vi "ResultSolver.vi"(8 "error in (no error)":errorcluster, 9 "Conf. Gral.":T2, 10 "Tipo de Med":T1, 11 "Array":sgl[](array[numeric])) -> (0 "error out":errorcluster, 3 "Result":sgl)   [LabVIEW 2014, in "MathLoop.lvlib"]
doc: "Calcula todos los resultados de Tiempo Real y Post-proceso."
uses:
  MathLoop.lvlib
  TypeDefs/Conf. Gral.ctl
  TypeDefs/typeMed.ctl
  <vilib>/Analysis/baseanly.llb/Mean (DBL).vi
  <vilib>/Analysis/2dsp.llb/Real FFT.vi
  <vilib>/Analysis/2dsp.llb/Inverse Complex FFT.vi
  <vilib>/Analysis/NI_AALBase.lvlib
  <vilib>/Analysis/NI_AALPro.lvlib
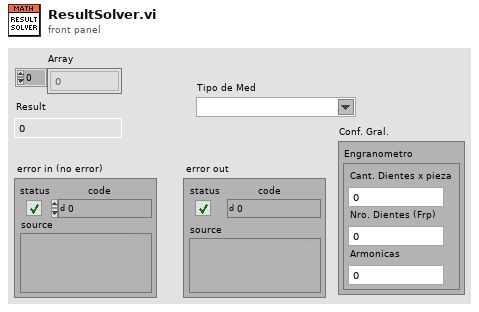
[diagram p1: front panel]
types:
  T1 = typedef "MathLoop.lvlib/typeMed.ctl" = string
  T2 = typedef "MathLoop.lvlib/Conf. Gral.ctl" = cluster{"Engranometro":cluster{"Cant. Dientes x pieza":i32, "Nro. Dientes (Frp)":i32, "Armonicas":i32}}
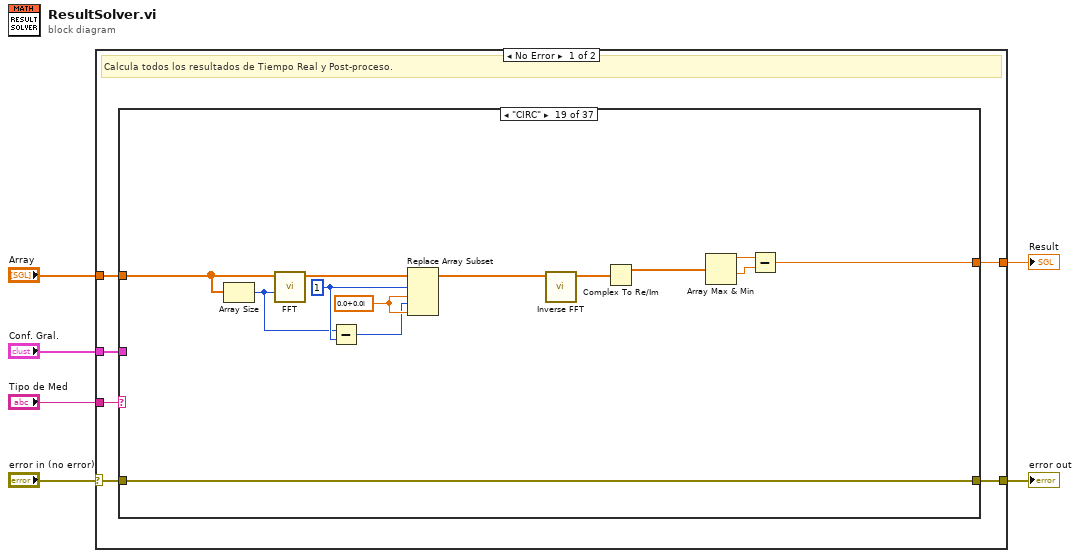
[diagram p0: block diagram]
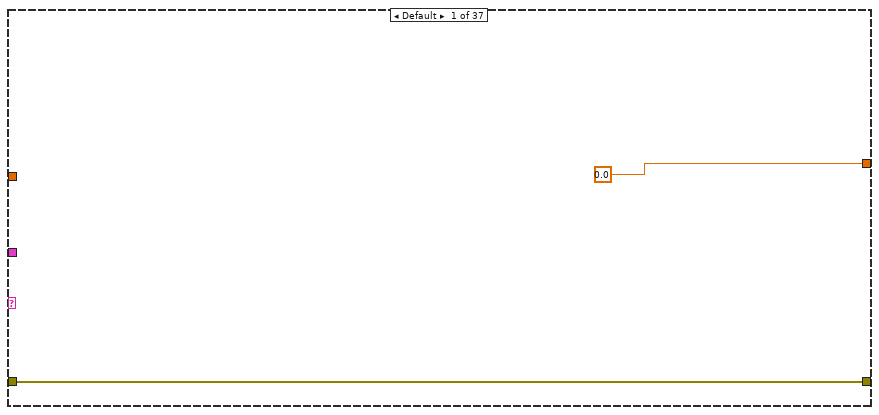
[diagram p2: hidden frame]
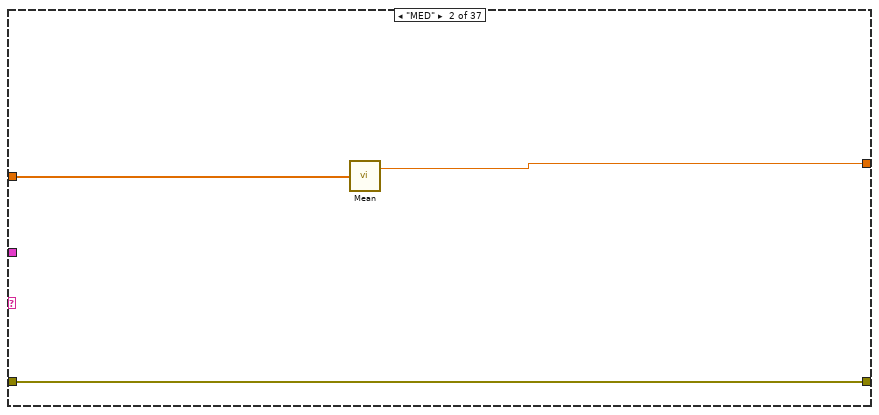
[diagram p3: hidden frame]
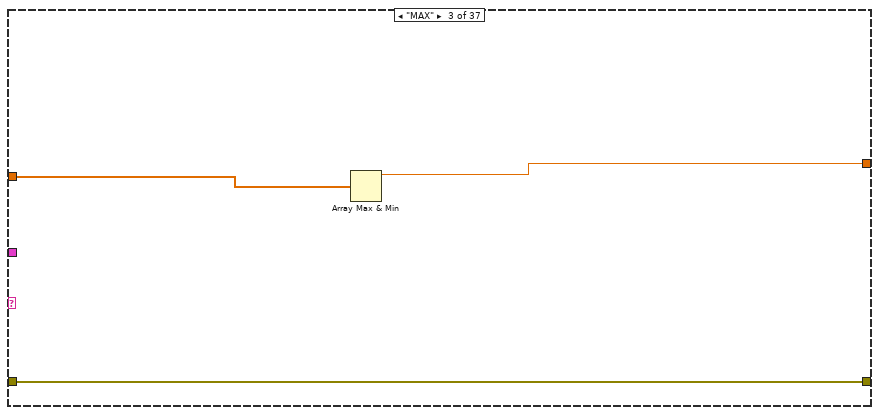
[diagram p4: hidden frame]
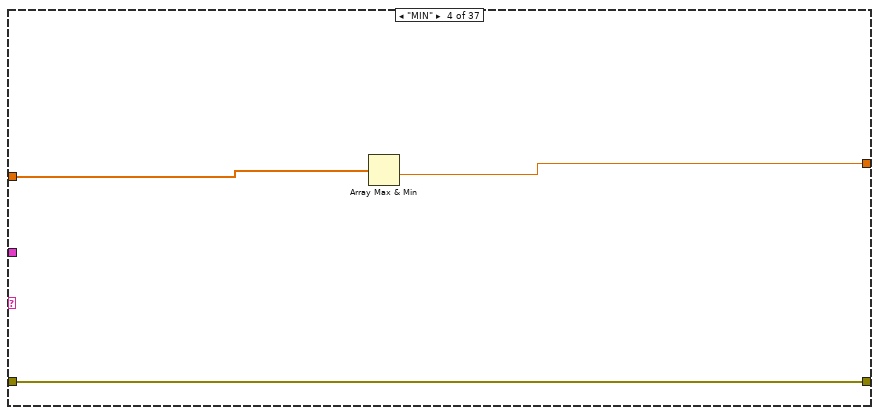
[diagram p5: hidden frame]
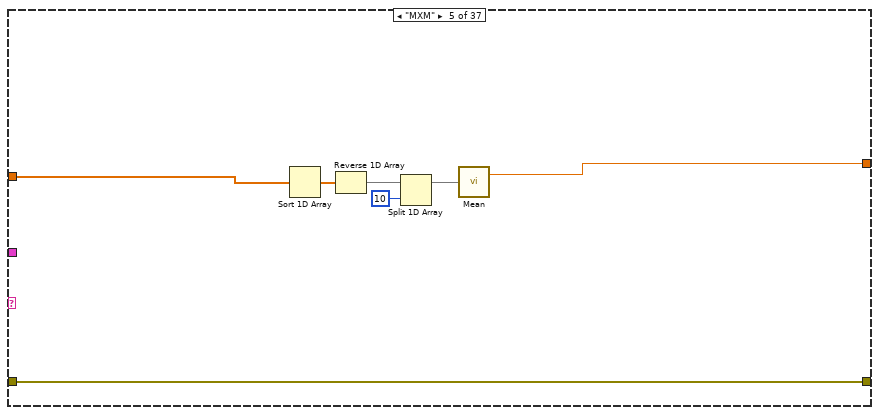
[diagram p6: hidden frame]
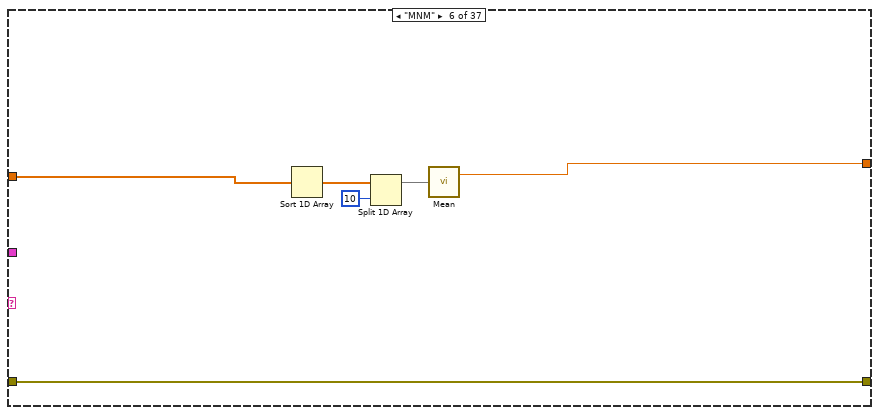
[diagram p7: hidden frame]
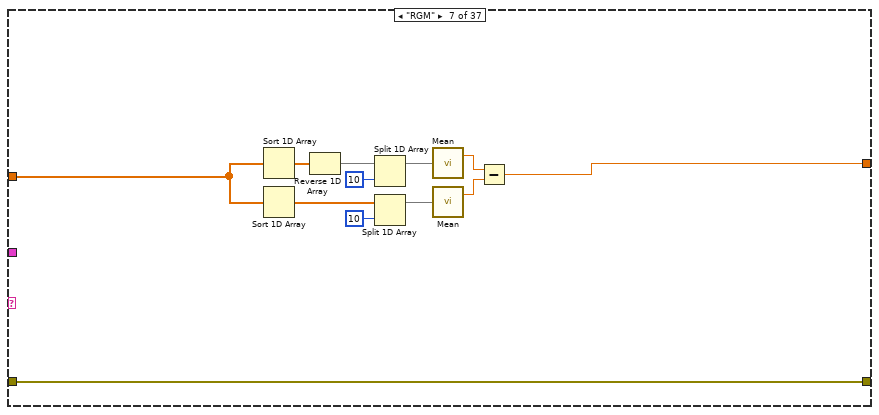
[diagram p8: hidden frame]
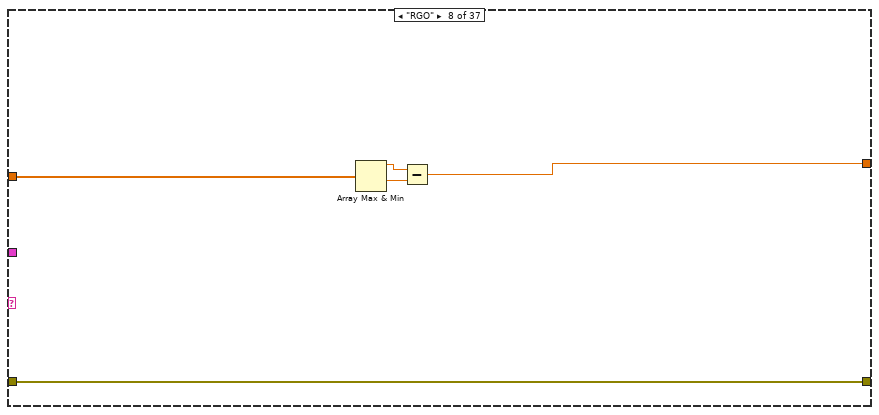
[diagram p9: hidden frame]
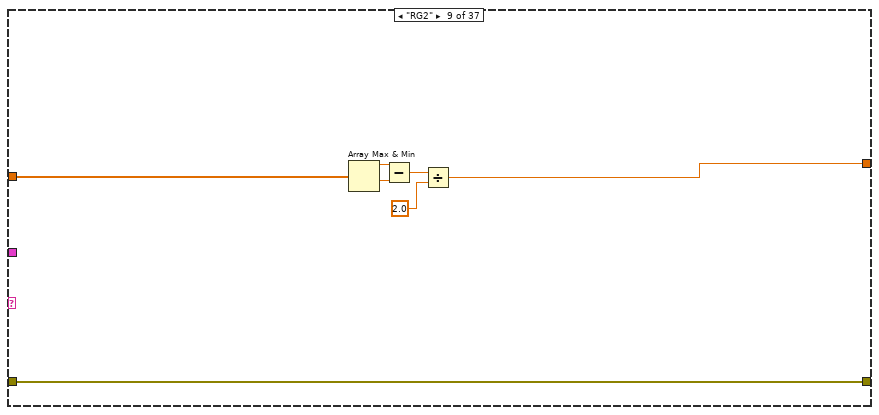
[diagram p10: hidden frame]
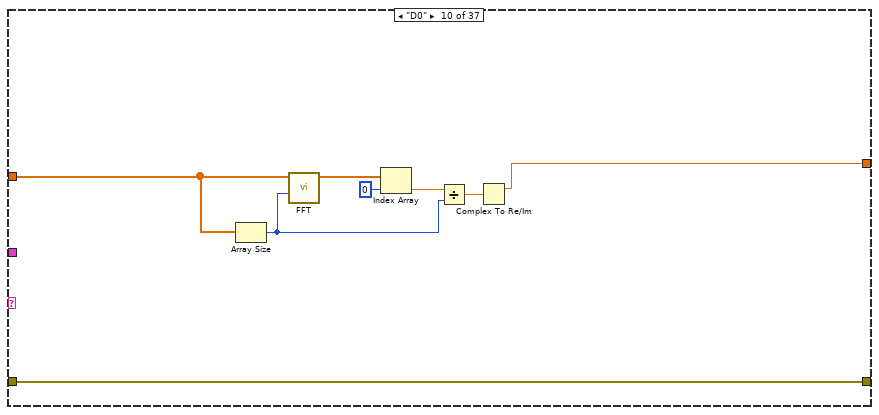
[diagram p11: hidden frame]
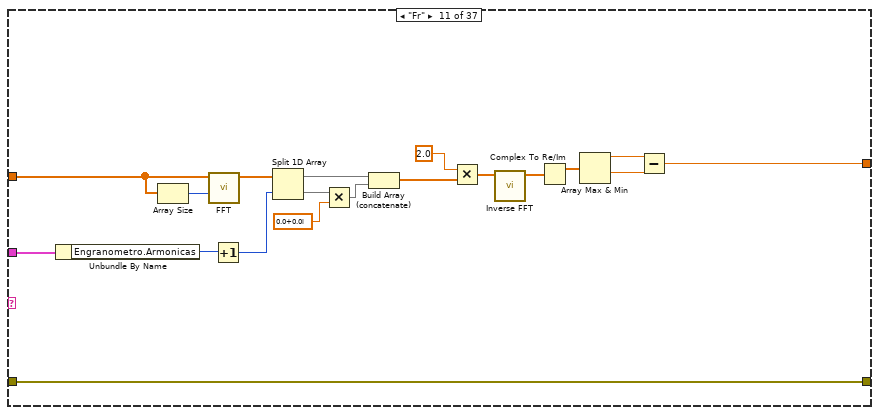
[diagram p12: hidden frame]
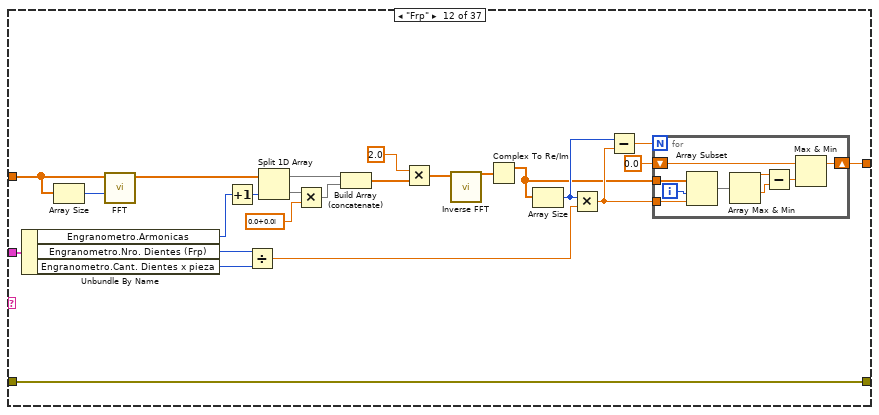
[diagram p13: hidden frame]
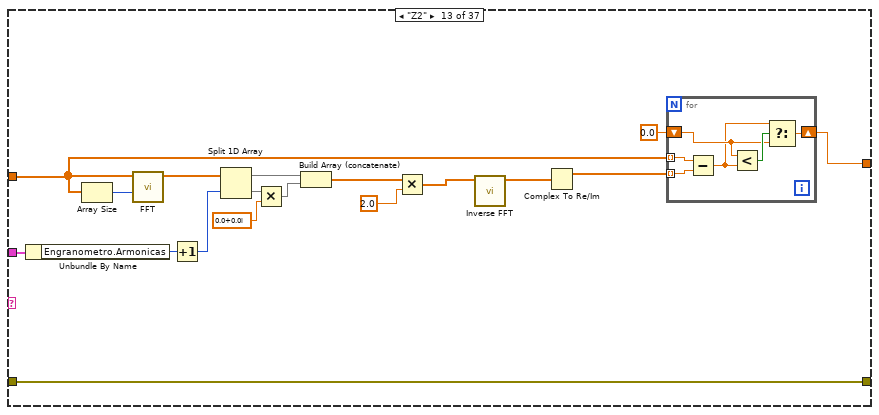
[diagram p14: hidden frame]
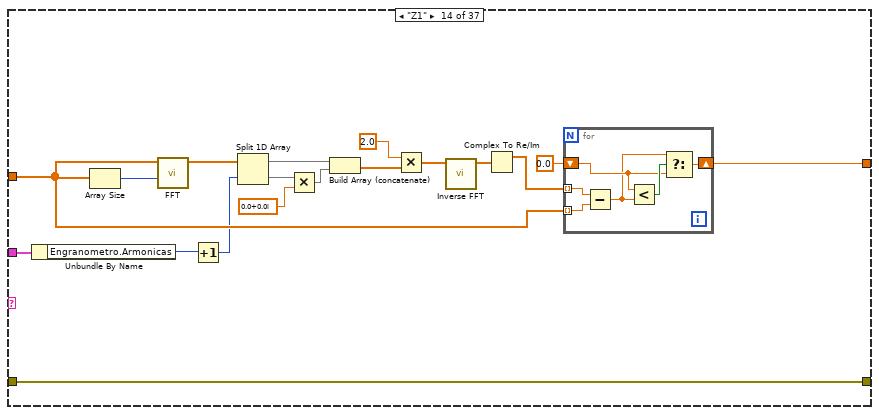
[diagram p15: hidden frame]
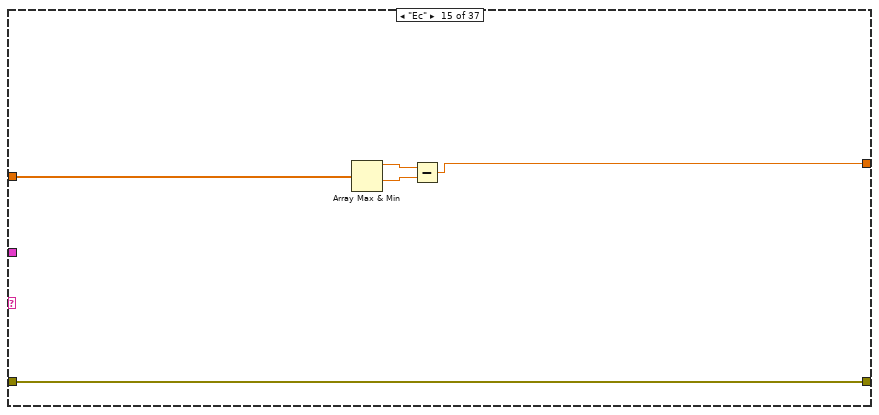
[diagram p16: hidden frame]
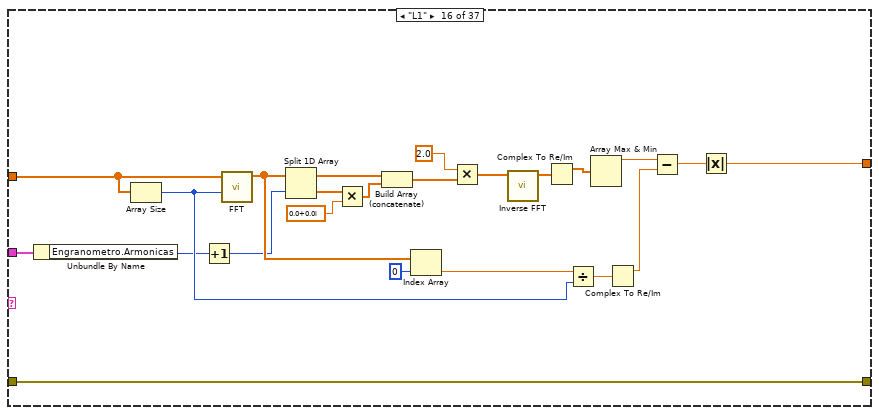
[diagram p17: hidden frame]
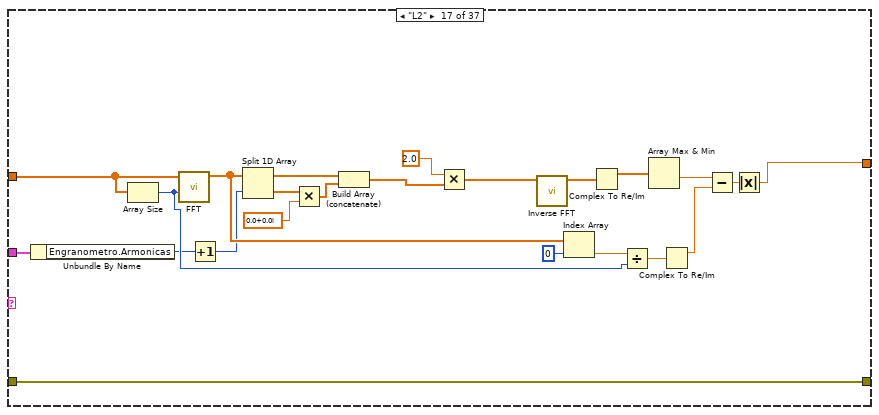
[diagram p18: hidden frame]
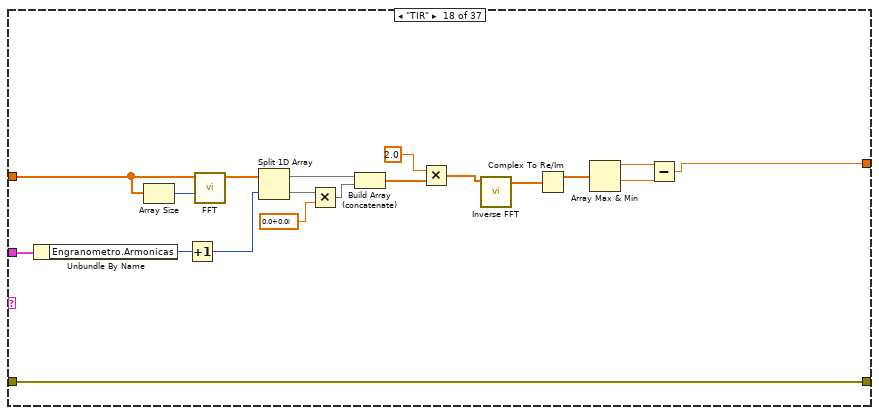
[diagram p19: hidden frame]
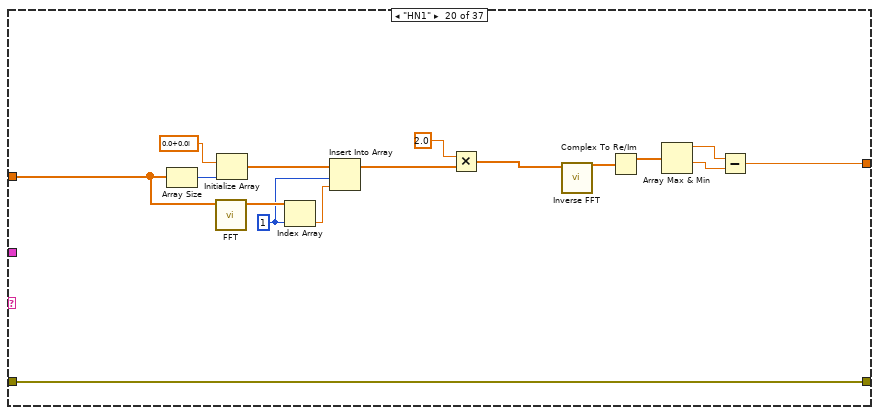
[diagram p20: hidden frame]
diagram:
  n1 = case shown="No Error" "error in (no error)" {
    selector: "error in (no error)" -> [w9 w561]
    tunnel: [w10 w561] -> w5
    tunnel: "Tipo de Med" -> [w12 _]
    tunnel: "Array" -> [w11 _]
    tunnel: [w7 0.0 ("mean")] -> w3
    tunnel: "Conf. Gral." -> [w8 _]
    frame No Error {
      # "Calcula todos los resultados de Tiempo Real y Post-proceso."
      n2 = case shown="\"CIRC\"" w12 {
        tunnel: w11 -> [_ w17 w20 w23 w25 w34 w40 w50 w59 w64 w86 w104 w130 w152 w172 w191 w214 w229 w247 w262 w274 w290 w306 w322 w338 w354 w370 w386 w402 w418 w434 w450 w466 w482 w498 w512 w554]
        tunnel: [0.0 ("mean") w16 w19 w22 w26 w33 w39 w51 w58 w61 w82 w95 w128 w153 w169 w181 w204 w228 w248 w258 w273 w289 w305 w321 w337 w353 w369 w385 w401 w417 w433 w449 w465 w481 w497 w510 w538] -> w7
        tunnel: [w14 w15 w18 w21 w24 w31 w38 w49 w54 w66 w87 w111 w138 w162 w173 w196 w219 w238 w251 w267 w283 w299 w315 w331 w347 w363 w379 w395 w411 w427 w443 w459 w475 w491 w507 w515 w559] -> w10
        tunnel: w9 -> [w14 w15 w18 w21 w24 w31 w38 w49 w54 w66 w87 w111 w138 w162 w173 w196 w219 w238 w251 w267 w283 w299 w315 w331 w347 w363 w379 w395 w411 w427 w443 w459 w475 w491 w507 w515 w559]
        tunnel: w8 -> [_ _ _ _ _ _ _ _ _ _ w81 w103 w131 w155 _ w190 w213 w227 _ _ _ _ _ _ _ _ _ _ _ _ _ _ _ _ _ w514 w555]
        frame Default {
        }
        frame "MED" {
          n3 = call-poly <vilib>:"Mean.vi"("X"=w17) -> ("mean"=w16:dbl)  [unwired: 1 out]
        }
        frame "MAX" {
          n4 = Array Max & Min(array=w20) -> (max value=w19:sgl)  [unwired: 3 out]
        }
        frame "MIN" {
          n5 = Array Max & Min(array=w23) -> (min value=w22:sgl)  [unwired: 3 out]
        }
        frame "MXM" {
          n6 = Sort 1D Array(array=w25) -> (sorted array=w28:sgl[])
          n7 = Reverse 1D Array(array=w28) -> (reversed array=w27:sgl[])
          n8 = Split 1D Array(array=w27, index=10) -> (first subarray=w29:sgl[])  [unwired: 1 out]
          n9 = call-poly <vilib>:"Mean.vi"("X"=w29) -> ("mean"=w26:dbl)  [unwired: 1 out]
        }
        frame "MNM" {
          n10 = Sort 1D Array(array=w34) -> (sorted array=w35:sgl[])
          n11 = Split 1D Array(array=w35, index=10) -> (first subarray=w36:sgl[])  [unwired: 1 out]
          n12 = call-poly <vilib>:"Mean.vi"("X"=w36) -> ("mean"=w33:dbl)  [unwired: 1 out]
        }
        frame "RGM" {
          n13 = Sort 1D Array(array=w40) -> (sorted array=w45:sgl[])
          n14 = Sort 1D Array(array=w40) -> (sorted array=w48:sgl[])
          n15 = Reverse 1D Array(array=w45) -> (reversed array=w46:sgl[])
          n16 = Split 1D Array(array=w46, index=10) -> (first subarray=w44:sgl[])  [unwired: 1 out]
          n17 = Split 1D Array(array=w48, index=10) -> (first subarray=w47:sgl[])  [unwired: 1 out]
          n18 = call-poly <vilib>:"Mean.vi"("X"=w44) -> ("mean"=w42:dbl)  [unwired: 1 out]
          n19 = call-poly <vilib>:"Mean.vi"("X"=w47) -> ("mean"=w41:dbl)  [unwired: 1 out]
          n20 = Subtract(x=w42, y=w41) -> (x-y=w39:dbl)
        }
        frame "RGO" {
          n21 = Array Max & Min(array=w50) -> (max value=w53:sgl, min value=w52:sgl)  [unwired: 2 out]
          n22 = Subtract(x=w53, y=w52) -> (x-y=w51:sgl)
        }
        frame "RG2" {
          n23 = Array Max & Min(array=w59) -> (max value=w56:sgl, min value=w55:sgl)  [unwired: 2 out]
          n24 = Subtract(x=w56, y=w55) -> (x-y=w57:sgl)
          n25 = Divide(x=w57, y=sgl 2.0) -> (x/y=w58:sgl)
        }
        frame "D0" {
          n26 = Array Size(array=w64) -> (size(s)=w63:i32)
          n27 = call-poly <vilib>:"FFT.vi"("FFT size"=w63, "X"=w64) -> ("FFT {X}"=w68:cdb[])  [unwired: 8 in, 1 out]
          n28 = Index Array(array=w68, index=0) -> (element=w62:cdb)
          n29 = Divide(x=w62, y=w63) -> (x/y=w65:cdb)
          n30 = Complex To Re/Im(x + iy=w65) -> (x=w61:dbl)  [unwired: 1 out]
        }
        frame "Fr" {
          n31 = Unbundle By Name(w81) -> ("Engranometro.Armonicas"=w73:i32)
          n32 = Array Size(array=w86) -> (size(s)=w85:i32)
          n33 = call-poly <vilib>:"FFT.vi"("FFT size"=w85, "X"=w86) -> ("FFT {X}"=w80:cdb[])  [unwired: 8 in, 1 out]
          n34 = Increment(x=w73) -> (x+1=w72:i32)
          n35 = Split 1D Array(array=w80, index=w72) -> (first subarray=w79:cdb[], second subarray=w76:cdb[])
          n36 = Multiply(x=w76, y=cdb 0.0+0.0i) -> (x*y=w77:cdb[])
          n37 = Build Array (concatenate)(w79, w77) -> (w70:cdb[])
          n38 = Multiply(x=2.0, y=w70) -> (x*y=w69:cdb[])
          n39 = call-poly <vilib>:"Inverse FFT.vi"("FFT {X}"=w69) -> ("X"=w75:cdb[])  [unwired: 9 in, 1 out]
          n40 = Complex To Re/Im(x + iy=w75) -> (x=w74:dbl[])  [unwired: 1 out]
          n41 = Array Max & Min(array=w74) -> (max value=w84:dbl, min value=w83:dbl)  [unwired: 2 out]
          n42 = Subtract(x=w84, y=w83) -> (x-y=w82:dbl)
        }
        frame "Frp" {
          n43 = Unbundle By Name(w103) -> ("Engranometro.Armonicas"=w91:i32, "Engranometro.Nro. Dientes (Frp)"=w98:i32, "Engranometro.Cant. Dientes x pieza"=w97:i32)
          n44 = Array Size(array=w104) -> (size(s)=w110:i32)
          n45 = call-poly <vilib>:"FFT.vi"("FFT size"=w110, "X"=w104) -> ("FFT {X}"=w109:cdb[])  [unwired: 8 in, 1 out]
          n46 = Increment(x=w91) -> (x+1=w92:i32)
          n47 = Divide(x=w98, y=w97) -> (x/y=w96:dbl)
          n48 = Split 1D Array(array=w109, index=w92) -> (first subarray=w108:cdb[], second subarray=w105:cdb[])
          n49 = Multiply(x=w105, y=cdb 0.0+0.0i) -> (x*y=w106:cdb[])
          n50 = Build Array (concatenate)(w108, w106) -> (w89:cdb[])
          n51 = Multiply(x=2.0, y=w89) -> (x*y=w88:cdb[])
          n52 = call-poly <vilib>:"Inverse FFT.vi"("FFT {X}"=w88) -> ("X"=w94:cdb[])  [unwired: 9 in, 1 out]
          n53 = Complex To Re/Im(x + iy=w94) -> (x=w93:dbl[])  [unwired: 1 out]
          n54 = Array Size(array=w93) -> (size(s)=w101:i32)
          n55 = Multiply(x=w101, y=w96) -> (x*y=w100:dbl)
          n56 = Subtract(x=w101, y=w100) -> (x-y=w99:dbl)
          n57 = for {
            N: w99 -> [_]
            tunnel: w93 -> [w114]
            tunnel: w100 -> [w113]
            shift-right: [w117] -> w95
            shift-left: 0.0 ("element") -> [w115]
            i -> [w112]
            n58 = Array Subset(array=w114, index=w112, length=w113) -> (w120:dbl[])
            n59 = Array Max & Min(array=w120) -> (max value=w119:dbl, min value=w118:dbl)  [unwired: 2 out]
            n60 = Subtract(x=w119, y=w118) -> (x-y=w116:dbl)
            n61 = Max & Min(x=w115, y=w116) -> (max(x,y)=w117:dbl)  [unwired: 1 out]
          }
        }
        frame "Z2" {
          n62 = Unbundle By Name(w131) -> ("Engranometro.Armonicas"=w125:i32)
          n63 = Array Size(array=w130) -> (size(s)=w137:i32)
          n64 = call-poly <vilib>:"FFT.vi"("FFT size"=w137, "X"=w130) -> ("FFT {X}"=w136:cdb[])  [unwired: 8 in, 1 out]
          n65 = Increment(x=w125) -> (x+1=w124:i32)
          n66 = Split 1D Array(array=w136, index=w124) -> (first subarray=w135:cdb[], second subarray=w132:cdb[])
          n67 = Multiply(x=w132, y=cdb 0.0+0.0i) -> (x*y=w133:cdb[])
          n68 = Build Array (concatenate)(w135, w133) -> (w121:cdb[])
          n69 = Multiply(x=w121, y=2.0 ("x")) -> (x*y=w122:cdb[])
          n70 = call-poly <vilib>:"Inverse FFT.vi"("FFT {X}"=w122) -> ("X"=w127:cdb[])  [unwired: 9 in, 1 out]
          n71 = Complex To Re/Im(x + iy=w127) -> (x=w126:dbl[])  [unwired: 1 out]
          n72 = for {
            tunnel: w126 -> [w143] mode=indexing
            tunnel: w130 -> [w144] mode=indexing
            shift-right: [w139] -> w128
            shift-left: 0.0 -> [w141]
            n73 = Subtract(x=w144, y=w143) -> (x-y=w140:dbl)
            n74 = Less?(x=w141, y=w140) -> (x < y?=w142:bool)
            n75 = Select(t=w140, s=w142, f=w141) -> (s? t:f=w139:dbl)
          }
        }
        frame "Z1" {
          n76 = Unbundle By Name(w155) -> ("Engranometro.Armonicas"=w149:i32)
          n77 = Array Size(array=w152) -> (size(s)=w161:i32)
          n78 = call-poly <vilib>:"FFT.vi"("FFT size"=w161, "X"=w152) -> ("FFT {X}"=w160:cdb[])  [unwired: 8 in, 1 out]
          n79 = Increment(x=w149) -> (x+1=w148:i32)
          n80 = Split 1D Array(array=w160, index=w148) -> (first subarray=w159:cdb[], second subarray=w156:cdb[])
          n81 = Multiply(x=w156, y=cdb 0.0+0.0i) -> (x*y=w157:cdb[])
          n82 = Build Array (concatenate)(w159, w157) -> (w146:cdb[])
          n83 = Multiply(x=2.0, y=w146) -> (x*y=w145:cdb[])
          n84 = call-poly <vilib>:"Inverse FFT.vi"("FFT {X}"=w145) -> ("X"=w151:cdb[])  [unwired: 9 in, 1 out]
          n85 = Complex To Re/Im(x + iy=w151) -> (x=w150:dbl[])  [unwired: 1 out]
          n86 = for {
            tunnel: w152 -> [w167] mode=indexing
            tunnel: w150 -> [w168] mode=indexing
            shift-right: [w163] -> w153
            shift-left: 0.0 -> [w165]
            n87 = Subtract(x=w168, y=w167) -> (x-y=w164:dbl)
            n88 = Less?(x=w165, y=w164) -> (x < y?=w166:bool)
            n89 = Select(t=w164, s=w166, f=w165) -> (s? t:f=w163:dbl)
          }
        }
        frame "Ec" {
          n90 = Array Max & Min(array=w172) -> (max value=w171:sgl, min value=w170:sgl)  [unwired: 2 out]
          n91 = Subtract(x=w171, y=w170) -> (x-y=w169:sgl)
        }
        frame "L1" {
          n92 = Unbundle By Name(w190) -> ("Engranometro.Armonicas"=w178:i32)
          n93 = Array Size(array=w191) -> (size(s)=w184:i32)
          n94 = Increment(x=w178) -> (x+1=w177:i32)
          n95 = call-poly <vilib>:"FFT.vi"("FFT size"=w184, "X"=w191) -> ("FFT {X}"=w185:cdb[])  [unwired: 8 in, 1 out]
          n96 = Split 1D Array(array=w185, index=w177) -> (first subarray=w195:cdb[], second subarray=w192:cdb[])
          n97 = Multiply(x=w192, y=cdb 0.0+0.0i) -> (x*y=w193:cdb[])
          n98 = Build Array (concatenate)(w195, w193) -> (w175:cdb[])
          n99 = Index Array(array=w185, index=0) -> (element=w186:cdb)
          n100 = Multiply(x=2.0, y=w175) -> (x*y=w174:cdb[])
          n101 = call-poly <vilib>:"Inverse FFT.vi"("FFT {X}"=w174) -> ("X"=w180:cdb[])  [unwired: 9 in, 1 out]
          n102 = Complex To Re/Im(x + iy=w180) -> (x=w179:dbl[])  [unwired: 1 out]
          n103 = Divide(x=w186, y=w184) -> (x/y=w187:cdb)
          n104 = Array Max & Min(array=w179) -> (max value=w189:dbl)  [unwired: 3 out]
          n105 = Complex To Re/Im(x + iy=w187) -> (x=w183:dbl)  [unwired: 1 out]
          n106 = Subtract(x=w189, y=w183) -> (x-y=w182:dbl)
          n107 = Absolute Value(x=w182) -> (abs(x)=w181:dbl)
        }
        frame "L2" {
          n108 = Unbundle By Name(w213) -> ("Engranometro.Armonicas"=w200:i32)
          n109 = Array Size(array=w214) -> (size(s)=w206:i32)
          n110 = call-poly <vilib>:"FFT.vi"("FFT size"=w206, "X"=w214) -> ("FFT {X}"=w207:cdb[])  [unwired: 8 in, 1 out]
          n111 = Increment(x=w200) -> (x+1=w201:i32)
          n112 = Split 1D Array(array=w207, index=w201) -> (first subarray=w218:cdb[], second subarray=w215:cdb[])
          n113 = Multiply(x=w215, y=cdb 0.0+0.0i) -> (x*y=w216:cdb[])
          n114 = Build Array (concatenate)(w218, w216) -> (w198:cdb[])
          n115 = Multiply(x=2.0, y=w198) -> (x*y=w197:cdb[])
          n116 = call-poly <vilib>:"Inverse FFT.vi"("FFT {X}"=w197) -> ("X"=w203:cdb[])  [unwired: 9 in, 1 out]
          n117 = Index Array(array=w207, index=0) -> (element=w210:cdb)
          n118 = Complex To Re/Im(x + iy=w203) -> (x=w202:dbl[])  [unwired: 1 out]
          n119 = Divide(x=w210, y=w206) -> (x/y=w211:cdb)
          n120 = Array Max & Min(array=w202) -> (min value=w209:dbl)  [unwired: 3 out]
          n121 = Complex To Re/Im(x + iy=w211) -> (x=w208:dbl)  [unwired: 1 out]
          n122 = Subtract(x=w209, y=w208) -> (x-y=w205:dbl)
          n123 = Absolute Value(x=w205) -> (abs(x)=w204:dbl)
        }
        frame "TIR" {
          n124 = Unbundle By Name(w227) -> ("Engranometro.Armonicas"=w224:i32)
          n125 = Array Size(array=w229) -> (size(s)=w237:i32)
          n126 = Increment(x=w224) -> (x+1=w223:i32)
          n127 = call-poly <vilib>:"FFT.vi"("FFT size"=w237, "X"=w229) -> ("FFT {X}"=w234:cdb[])  [unwired: 8 in, 1 out]
          n128 = Split 1D Array(array=w234, index=w223) -> (first subarray=w233:cdb[], second subarray=w230:cdb[])
          n129 = Multiply(x=w230, y=cdb 0.0+0.0i) -> (x*y=w231:cdb[])
          n130 = Build Array (concatenate)(w233, w231) -> (w221:cdb[])
          n131 = Multiply(x=2.0, y=w221) -> (x*y=w220:cdb[])
          n132 = call-poly <vilib>:"Inverse FFT.vi"("FFT {X}"=w220) -> ("X"=w226:cdb[])  [unwired: 9 in, 1 out]
          n133 = Complex To Re/Im(x + iy=w226) -> (x=w225:dbl[])  [unwired: 1 out]
          n134 = Array Max & Min(array=w225) -> (max value=w236:dbl, min value=w235:dbl)  [unwired: 2 out]
          n135 = Subtract(x=w236, y=w235) -> (x-y=w228:dbl)
        }
        frame "CIRC" {
          w244 = cdb 0.0+0.0i ("new element/subarray")
          w240 = 1 ("index")
          n136 = Array Size(array=w247) -> (size(s)=w239:i32)
          n137 = call-poly <vilib>:"FFT.vi"("FFT size"=w239, "X"=w247) -> ("FFT {X}"=w242:cdb[])  [unwired: 8 in, 1 out]
          n138 = Subtract(x=w239, y=w240) -> (x-y=w243:i32)
          n139 = Replace Array Subset(array=w242, new element #1=w244, index #1=w240, new element #2=w244, index #2=w243) -> (w241:cdb[])
          n140 = call-poly <vilib>:"Inverse FFT.vi"("FFT {X}"=w241) -> ("X"=w246:cdb[])  [unwired: 9 in, 1 out]
          n141 = Complex To Re/Im(x + iy=w246) -> (x=w245:dbl[])  [unwired: 1 out]
          n142 = Array Max & Min(array=w245) -> (max value=w250:dbl, min value=w249:dbl)  [unwired: 2 out]
          n143 = Subtract(x=w250, y=w249) -> (x-y=w248:dbl)
        }
        frame "HN1" {
          w261 = 1 ("index")
          n144 = Array Size(array=w262) -> (size(s)=w263:i32)
          n145 = call-poly <vilib>:"FFT.vi"("X"=w262) -> ("FFT {X}"=w264:cdb[])  [unwired: 9 in, 1 out]
          n146 = Initialize Array(cdb 0.0+0.0i ("element"), w263) -> (w266:cdb[])
          n147 = Index Array(array=w264, index=w261) -> (element=w257:cdb)
          n148 = Insert Into Array(array=w266, index=w261, new element=w257) -> (w253:cdb[])
          n149 = Multiply(x=2.0, y=w253) -> (x*y=w252:cdb[])
          n150 = call-poly <vilib>:"Inverse FFT.vi"("FFT {X}"=w252) -> ("X"=w256:cdb[])  [unwired: 9 in, 1 out]
          n151 = Complex To Re/Im(x + iy=w256) -> (x=w255:dbl[])  [unwired: 1 out]
          n152 = Array Max & Min(array=w255) -> (max value=w260:dbl, min value=w259:dbl)  [unwired: 2 out]
          n153 = Subtract(x=w260, y=w259) -> (x-y=w258:dbl)
        }
        frame "HN2" {
          w279 = 2 ("index")
          n154 = Array Size(array=w274) -> (size(s)=w278:i32)
          n155 = call-poly <vilib>:"FFT.vi"("X"=w274) -> ("FFT {X}"=w277:cdb[])  [unwired: 9 in, 1 out]
          n156 = Initialize Array(cdb 0.0+0.0i ("element"), w278) -> (w275:cdb[])
          n157 = Index Array(array=w277, index=w279) -> (element=w282:cdb)
          n158 = Insert Into Array(array=w275, index=w279, new element=w282) -> (w269:cdb[])
          n159 = Multiply(x=2.0, y=w269) -> (x*y=w268:cdb[])
          n160 = call-poly <vilib>:"Inverse FFT.vi"("FFT {X}"=w268) -> ("X"=w272:cdb[])  [unwired: 9 in, 1 out]
          n161 = Complex To Re/Im(x + iy=w272) -> (x=w271:dbl[])  [unwired: 1 out]
          n162 = Array Max & Min(array=w271) -> (max value=w280:dbl, min value=w281:dbl)  [unwired: 2 out]
          n163 = Subtract(x=w280, y=w281) -> (x-y=w273:dbl)
        }
        frame "HN3" {
          w295 = 3 ("index")
          n164 = Array Size(array=w290) -> (size(s)=w294:i32)
          n165 = call-poly <vilib>:"FFT.vi"("X"=w290) -> ("FFT {X}"=w293:cdb[])  [unwired: 9 in, 1 out]
          n166 = Initialize Array(cdb 0.0+0.0i ("element"), w294) -> (w291:cdb[])
          n167 = Index Array(array=w293, index=w295) -> (element=w298:cdb)
          n168 = Insert Into Array(array=w291, index=w295, new element=w298) -> (w285:cdb[])
          n169 = Multiply(x=2.0, y=w285) -> (x*y=w284:cdb[])
          n170 = call-poly <vilib>:"Inverse FFT.vi"("FFT {X}"=w284) -> ("X"=w288:cdb[])  [unwired: 9 in, 1 out]
          n171 = Complex To Re/Im(x + iy=w288) -> (x=w287:dbl[])  [unwired: 1 out]
          n172 = Array Max & Min(array=w287) -> (max value=w296:dbl, min value=w297:dbl)  [unwired: 2 out]
          n173 = Subtract(x=w296, y=w297) -> (x-y=w289:dbl)
        }
        frame "HN4" {
          w311 = 4 ("index")
          n174 = Array Size(array=w306) -> (size(s)=w310:i32)
          n175 = call-poly <vilib>:"FFT.vi"("X"=w306) -> ("FFT {X}"=w309:cdb[])  [unwired: 9 in, 1 out]
          n176 = Initialize Array(cdb 0.0+0.0i ("element"), w310) -> (w307:cdb[])
          n177 = Index Array(array=w309, index=w311) -> (element=w314:cdb)
          n178 = Insert Into Array(array=w307, index=w311, new element=w314) -> (w301:cdb[])
          n179 = Multiply(x=2.0, y=w301) -> (x*y=w300:cdb[])
          n180 = call-poly <vilib>:"Inverse FFT.vi"("FFT {X}"=w300) -> ("X"=w304:cdb[])  [unwired: 9 in, 1 out]
          n181 = Complex To Re/Im(x + iy=w304) -> (x=w303:dbl[])  [unwired: 1 out]
          n182 = Array Max & Min(array=w303) -> (max value=w312:dbl, min value=w313:dbl)  [unwired: 2 out]
          n183 = Subtract(x=w312, y=w313) -> (x-y=w305:dbl)
        }
        frame "HN5" {
          w327 = 5 ("index")
          n184 = Array Size(array=w322) -> (size(s)=w326:i32)
          n185 = call-poly <vilib>:"FFT.vi"("X"=w322) -> ("FFT {X}"=w325:cdb[])  [unwired: 9 in, 1 out]
          n186 = Initialize Array(cdb 0.0+0.0i ("element"), w326) -> (w323:cdb[])
          n187 = Index Array(array=w325, index=w327) -> (element=w330:cdb)
          n188 = Insert Into Array(array=w323, index=w327, new element=w330) -> (w317:cdb[])
          n189 = Multiply(x=2.0, y=w317) -> (x*y=w316:cdb[])
          n190 = call-poly <vilib>:"Inverse FFT.vi"("FFT {X}"=w316) -> ("X"=w320:cdb[])  [unwired: 9 in, 1 out]
          n191 = Complex To Re/Im(x + iy=w320) -> (x=w319:dbl[])  [unwired: 1 out]
          n192 = Array Max & Min(array=w319) -> (max value=w328:dbl, min value=w329:dbl)  [unwired: 2 out]
          n193 = Subtract(x=w328, y=w329) -> (x-y=w321:dbl)
        }
        frame "HN6" {
          w343 = 6 ("index")
          n194 = Array Size(array=w338) -> (size(s)=w342:i32)
          n195 = call-poly <vilib>:"FFT.vi"("X"=w338) -> ("FFT {X}"=w341:cdb[])  [unwired: 9 in, 1 out]
          n196 = Initialize Array(cdb 0.0+0.0i ("element"), w342) -> (w339:cdb[])
          n197 = Index Array(array=w341, index=w343) -> (element=w346:cdb)
          n198 = Insert Into Array(array=w339, index=w343, new element=w346) -> (w333:cdb[])
          n199 = Multiply(x=2.0, y=w333) -> (x*y=w332:cdb[])
          n200 = call-poly <vilib>:"Inverse FFT.vi"("FFT {X}"=w332) -> ("X"=w336:cdb[])  [unwired: 9 in, 1 out]
          n201 = Complex To Re/Im(x + iy=w336) -> (x=w335:dbl[])  [unwired: 1 out]
          n202 = Array Max & Min(array=w335) -> (max value=w344:dbl, min value=w345:dbl)  [unwired: 2 out]
          n203 = Subtract(x=w344, y=w345) -> (x-y=w337:dbl)
        }
        frame "HN7" {
          w359 = 7 ("index")
          n204 = Array Size(array=w354) -> (size(s)=w358:i32)
          n205 = call-poly <vilib>:"FFT.vi"("X"=w354) -> ("FFT {X}"=w357:cdb[])  [unwired: 9 in, 1 out]
          n206 = Initialize Array(cdb 0.0+0.0i ("element"), w358) -> (w355:cdb[])
          n207 = Index Array(array=w357, index=w359) -> (element=w362:cdb)
          n208 = Insert Into Array(array=w355, index=w359, new element=w362) -> (w349:cdb[])
          n209 = Multiply(x=2.0, y=w349) -> (x*y=w348:cdb[])
          n210 = call-poly <vilib>:"Inverse FFT.vi"("FFT {X}"=w348) -> ("X"=w352:cdb[])  [unwired: 9 in, 1 out]
          n211 = Complex To Re/Im(x + iy=w352) -> (x=w351:dbl[])  [unwired: 1 out]
          n212 = Array Max & Min(array=w351) -> (max value=w360:dbl, min value=w361:dbl)  [unwired: 2 out]
          n213 = Subtract(x=w360, y=w361) -> (x-y=w353:dbl)
        }
        frame "HN8" {
          w375 = 8 ("index")
          n214 = Array Size(array=w370) -> (size(s)=w374:i32)
          n215 = call-poly <vilib>:"FFT.vi"("X"=w370) -> ("FFT {X}"=w373:cdb[])  [unwired: 9 in, 1 out]
          n216 = Initialize Array(cdb 0.0+0.0i ("element"), w374) -> (w371:cdb[])
          n217 = Index Array(array=w373, index=w375) -> (element=w378:cdb)
          n218 = Insert Into Array(array=w371, index=w375, new element=w378) -> (w365:cdb[])
          n219 = Multiply(x=2.0, y=w365) -> (x*y=w364:cdb[])
          n220 = call-poly <vilib>:"Inverse FFT.vi"("FFT {X}"=w364) -> ("X"=w368:cdb[])  [unwired: 9 in, 1 out]
          n221 = Complex To Re/Im(x + iy=w368) -> (x=w367:dbl[])  [unwired: 1 out]
          n222 = Array Max & Min(array=w367) -> (max value=w376:dbl, min value=w377:dbl)  [unwired: 2 out]
          n223 = Subtract(x=w376, y=w377) -> (x-y=w369:dbl)
        }
        frame "HN9" {
          w391 = 9 ("index")
          n224 = Array Size(array=w386) -> (size(s)=w390:i32)
          n225 = call-poly <vilib>:"FFT.vi"("X"=w386) -> ("FFT {X}"=w389:cdb[])  [unwired: 9 in, 1 out]
          n226 = Initialize Array(cdb 0.0+0.0i ("element"), w390) -> (w387:cdb[])
          n227 = Index Array(array=w389, index=w391) -> (element=w394:cdb)
          n228 = Insert Into Array(array=w387, index=w391, new element=w394) -> (w381:cdb[])
          n229 = Multiply(x=2.0, y=w381) -> (x*y=w380:cdb[])
          n230 = call-poly <vilib>:"Inverse FFT.vi"("FFT {X}"=w380) -> ("X"=w384:cdb[])  [unwired: 9 in, 1 out]
          n231 = Complex To Re/Im(x + iy=w384) -> (x=w383:dbl[])  [unwired: 1 out]
          n232 = Array Max & Min(array=w383) -> (max value=w392:dbl, min value=w393:dbl)  [unwired: 2 out]
          n233 = Subtract(x=w392, y=w393) -> (x-y=w385:dbl)
        }
        frame "HN10" {
          w407 = 10 ("index")
          n234 = Array Size(array=w402) -> (size(s)=w406:i32)
          n235 = call-poly <vilib>:"FFT.vi"("X"=w402) -> ("FFT {X}"=w405:cdb[])  [unwired: 9 in, 1 out]
          n236 = Initialize Array(cdb 0.0+0.0i ("element"), w406) -> (w403:cdb[])
          n237 = Index Array(array=w405, index=w407) -> (element=w410:cdb)
          n238 = Insert Into Array(array=w403, index=w407, new element=w410) -> (w397:cdb[])
          n239 = Multiply(x=2.0, y=w397) -> (x*y=w396:cdb[])
          n240 = call-poly <vilib>:"Inverse FFT.vi"("FFT {X}"=w396) -> ("X"=w400:cdb[])  [unwired: 9 in, 1 out]
          n241 = Complex To Re/Im(x + iy=w400) -> (x=w399:dbl[])  [unwired: 1 out]
          n242 = Array Max & Min(array=w399) -> (max value=w408:dbl, min value=w409:dbl)  [unwired: 2 out]
          n243 = Subtract(x=w408, y=w409) -> (x-y=w401:dbl)
        }
        frame "HN11" {
          w423 = 11 ("index")
          n244 = Array Size(array=w418) -> (size(s)=w422:i32)
          n245 = call-poly <vilib>:"FFT.vi"("X"=w418) -> ("FFT {X}"=w421:cdb[])  [unwired: 9 in, 1 out]
          n246 = Initialize Array(cdb 0.0+0.0i ("element"), w422) -> (w419:cdb[])
          n247 = Index Array(array=w421, index=w423) -> (element=w426:cdb)
          n248 = Insert Into Array(array=w419, index=w423, new element=w426) -> (w413:cdb[])
          n249 = Multiply(x=2.0, y=w413) -> (x*y=w412:cdb[])
          n250 = call-poly <vilib>:"Inverse FFT.vi"("FFT {X}"=w412) -> ("X"=w416:cdb[])  [unwired: 9 in, 1 out]
          n251 = Complex To Re/Im(x + iy=w416) -> (x=w415:dbl[])  [unwired: 1 out]
          n252 = Array Max & Min(array=w415) -> (max value=w424:dbl, min value=w425:dbl)  [unwired: 2 out]
          n253 = Subtract(x=w424, y=w425) -> (x-y=w417:dbl)
        }
        frame "HN12" {
          w439 = 12 ("index")
          n254 = Array Size(array=w434) -> (size(s)=w438:i32)
          n255 = call-poly <vilib>:"FFT.vi"("X"=w434) -> ("FFT {X}"=w437:cdb[])  [unwired: 9 in, 1 out]
          n256 = Initialize Array(cdb 0.0+0.0i ("element"), w438) -> (w435:cdb[])
          n257 = Index Array(array=w437, index=w439) -> (element=w442:cdb)
          n258 = Insert Into Array(array=w435, index=w439, new element=w442) -> (w429:cdb[])
          n259 = Multiply(x=2.0, y=w429) -> (x*y=w428:cdb[])
          n260 = call-poly <vilib>:"Inverse FFT.vi"("FFT {X}"=w428) -> ("X"=w432:cdb[])  [unwired: 9 in, 1 out]
          n261 = Complex To Re/Im(x + iy=w432) -> (x=w431:dbl[])  [unwired: 1 out]
          n262 = Array Max & Min(array=w431) -> (max value=w440:dbl, min value=w441:dbl)  [unwired: 2 out]
          n263 = Subtract(x=w440, y=w441) -> (x-y=w433:dbl)
        }
        frame "HN13" {
          w455 = 13 ("index")
          n264 = Array Size(array=w450) -> (size(s)=w454:i32)
          n265 = call-poly <vilib>:"FFT.vi"("X"=w450) -> ("FFT {X}"=w453:cdb[])  [unwired: 9 in, 1 out]
          n266 = Initialize Array(cdb 0.0+0.0i ("element"), w454) -> (w451:cdb[])
          n267 = Index Array(array=w453, index=w455) -> (element=w458:cdb)
          n268 = Insert Into Array(array=w451, index=w455, new element=w458) -> (w445:cdb[])
          n269 = Multiply(x=2.0, y=w445) -> (x*y=w444:cdb[])
          n270 = call-poly <vilib>:"Inverse FFT.vi"("FFT {X}"=w444) -> ("X"=w448:cdb[])  [unwired: 9 in, 1 out]
          n271 = Complex To Re/Im(x + iy=w448) -> (x=w447:dbl[])  [unwired: 1 out]
          n272 = Array Max & Min(array=w447) -> (max value=w456:dbl, min value=w457:dbl)  [unwired: 2 out]
          n273 = Subtract(x=w456, y=w457) -> (x-y=w449:dbl)
        }
        frame "HN14" {
          w471 = 14 ("index")
          n274 = Array Size(array=w466) -> (size(s)=w470:i32)
          n275 = call-poly <vilib>:"FFT.vi"("X"=w466) -> ("FFT {X}"=w469:cdb[])  [unwired: 9 in, 1 out]
          n276 = Initialize Array(cdb 0.0+0.0i ("element"), w470) -> (w467:cdb[])
          n277 = Index Array(array=w469, index=w471) -> (element=w474:cdb)
          n278 = Insert Into Array(array=w467, index=w471, new element=w474) -> (w461:cdb[])
          n279 = Multiply(x=2.0, y=w461) -> (x*y=w460:cdb[])
          n280 = call-poly <vilib>:"Inverse FFT.vi"("FFT {X}"=w460) -> ("X"=w464:cdb[])  [unwired: 9 in, 1 out]
          n281 = Complex To Re/Im(x + iy=w464) -> (x=w463:dbl[])  [unwired: 1 out]
          n282 = Array Max & Min(array=w463) -> (max value=w472:dbl, min value=w473:dbl)  [unwired: 2 out]
          n283 = Subtract(x=w472, y=w473) -> (x-y=w465:dbl)
        }
        frame "HN15" {
          w487 = 15 ("index")
          n284 = Array Size(array=w482) -> (size(s)=w486:i32)
          n285 = call-poly <vilib>:"FFT.vi"("X"=w482) -> ("FFT {X}"=w485:cdb[])  [unwired: 9 in, 1 out]
          n286 = Initialize Array(cdb 0.0+0.0i ("element"), w486) -> (w483:cdb[])
          n287 = Index Array(array=w485, index=w487) -> (element=w490:cdb)
          n288 = Insert Into Array(array=w483, index=w487, new element=w490) -> (w477:cdb[])
          n289 = Multiply(x=2.0, y=w477) -> (x*y=w476:cdb[])
          n290 = call-poly <vilib>:"Inverse FFT.vi"("FFT {X}"=w476) -> ("X"=w480:cdb[])  [unwired: 9 in, 1 out]
          n291 = Complex To Re/Im(x + iy=w480) -> (x=w479:dbl[])  [unwired: 1 out]
          n292 = Array Max & Min(array=w479) -> (max value=w488:dbl, min value=w489:dbl)  [unwired: 2 out]
          n293 = Subtract(x=w488, y=w489) -> (x-y=w481:dbl)
        }
        frame "HN16" {
          w503 = 16 ("index")
          n294 = Array Size(array=w498) -> (size(s)=w502:i32)
          n295 = call-poly <vilib>:"FFT.vi"("X"=w498) -> ("FFT {X}"=w501:cdb[])  [unwired: 9 in, 1 out]
          n296 = Initialize Array(cdb 0.0+0.0i ("element"), w502) -> (w499:cdb[])
          n297 = Index Array(array=w501, index=w503) -> (element=w506:cdb)
          n298 = Insert Into Array(array=w499, index=w503, new element=w506) -> (w493:cdb[])
          n299 = Multiply(x=2.0, y=w493) -> (x*y=w492:cdb[])
          n300 = call-poly <vilib>:"Inverse FFT.vi"("FFT {X}"=w492) -> ("X"=w496:cdb[])  [unwired: 9 in, 1 out]
          n301 = Complex To Re/Im(x + iy=w496) -> (x=w495:dbl[])  [unwired: 1 out]
          n302 = Array Max & Min(array=w495) -> (max value=w504:dbl, min value=w505:dbl)  [unwired: 2 out]
          n303 = Subtract(x=w504, y=w505) -> (x-y=w497:dbl)
        }
        frame "Fi" {
          n304 = Unbundle By Name(w514) -> ("Engranometro.Cant. Dientes x pieza"=w511:i32)
          n305 = Array Size(array=w512) -> (size(s)=w513:i32)
          n306 = Divide(x=w513, y=w511) -> (x/y=w509:dbl)
          n307 = for {
            N: w511 -> [_]
            shift-right: [w528] -> w510
            shift-left: sgl 0.0 -> [w527]
            shift-right: [w517] -> _
            shift-left: w512 -> [w530]
            tunnel: w509 -> [w519]
            n308 = Split 1D Array(array=w530, index=w519) -> (first subarray=w522:sgl[], second subarray=w517:sgl[])
            n309 = Multiply(x=1.4, y=w519) -> (x*y=w520:dbl)
            n310 = Subtract(x=w520, y=w519) -> (x-y=w518:dbl)
            n311 = Split 1D Array(array=w517, index=w518) -> (first subarray=w516:sgl[])  [unwired: 1 out]
            n312 = Build Array (concatenate)(w522, w516) -> (w523:sgl[])
            n313 = Array Max & Min(array=w523) -> (max value=w525:sgl, min value=w526:sgl)  [unwired: 2 out]
            n314 = Subtract(x=w525, y=w526) -> (x-y=w524:sgl)
            n315 = Less?(x=w524, y=w527) -> (x < y?=w529:bool)
            n316 = Select(t=w527, s=w529, f=w524) -> (s? t:f=w528:sgl)
          }
        }
        frame "Fk" {
          n317 = Unbundle By Name(w555) -> ("Engranometro.Cant. Dientes x pieza"=w534:i32)
          n318 = Array Size(array=w554) -> (size(s)=w556:i32)
          n319 = call-poly <vilib>:"FFT.vi"("FFT size"=w556, "X"=w554) -> ("FFT {X}"=w558:cdb[])  [unwired: 8 in, 1 out]
          n320 = Increment(x=w534) -> (x+1=w535:i32)
          n321 = Split 1D Array(array=w558, index=w535) -> (first subarray=w546:cdb[], second subarray=w553:cdb[])
          n322 = Array Size(array=w546) -> (size(s)=w548:i32)
          n323 = Subtract(x=w548, y=3) -> (x-y=w545:i32)
          n324 = Split 1D Array(array=w546, index=w545) -> (first subarray=w543:cdb[], second subarray=w542:cdb[])
          n325 = Split 1D Array(array=w553, index=2) -> (first subarray=w549:cdb[], second subarray=w551:cdb[])
          n326 = Multiply(x=cdb 0.0+0.0i, y=w543) -> (x*y=w541:cdb[])
          n327 = Multiply(x=w551, y=cdb 0.0+0.0i) -> (x*y=w550:cdb[])
          n328 = Build Array (concatenate)(w541, w542, w549, w550) -> (w532:cdb[])
          n329 = Multiply(x=2.0, y=w532) -> (x*y=w531:cdb[])
          n330 = call-poly <vilib>:"Inverse FFT.vi"("FFT {X}"=w531) -> ("X"=w537:cdb[])  [unwired: 9 in, 1 out]
          n331 = Complex To Re/Im(x + iy=w537) -> (x=w536:dbl[])  [unwired: 1 out]
          n332 = Array Max & Min(array=w536) -> (max value=w540:dbl, min value=w539:dbl)  [unwired: 2 out]
          n333 = Subtract(x=w540, y=w539) -> (x-y=w538:dbl)
        }
      }
    }
    frame Error {
    }
  }
  "error out" <- w5
  "Result" <- w3
